vi "phase_one.vi"() -> ()   [LabVIEW 2015]
uses:
  <vilib>/NXT/Block Support/NXT_InputPort.ctl
  <vilib>/NXT/Block Support/NXT_OutputPort.ctl
  <vilib>/NXT/Dual Mode Library/Sound/PlayD.vi
  <vilib>/NXT/Dual Mode Library/Display/clearDisplay.vi
  <vilib>/NXT/Dual Mode Library/Display/drawText.vi
  <vilib>/NXT/Dual Mode Library/Waits/Wait_Num.vi
  <vilib>/NXT/Dual Mode Library/Waits/Wait_Touch.vi
  <vilib>/NXT/Dual Mode Library/Sensors/EV3_Touch_Reset.vi
  <vilib>/NXT/Dual Mode Library/Sensors/Touch_Count.vi
  <vilib>/NXT/Dual Mode Library/Display/drawNumber.vi
  <vilib>/NXT/NXTIO Xnodes/NXTIONodeSubVIs/NXTMotorRunDistance.vi
  <vilib>/NXT/Dual Mode Library/Sensors/EV3_Color_Reflect.vi
  <vilib>/NXT/Dual Mode Library/Display/drawNumber_float.vi
  global1.vi
  <vilib>/NXT/NXTIO Xnodes/AddressXNode/NXTIOAddress.xnode
  <vilib>/NXT/NXTIO Xnodes/NXTIOXNode/NXTIO.xnode
  <vilib>/NXT/Subs/LVHSConnector.ctl
  <vilib>/NXT/LegoClasses/BrickReference/BrickReference.lvclass
panel:
  out "4: Compound 2":string
  out "4: Compound 1":string
  out "3: Compound 1":string
  out "3: Compound 2":string
  out "2: Compound 2":string
  out "1: Compoud 2":string
  out "2: Compound 1":string
  out "1: Compound 1":string
  out "Done with Phase One?":bool
  out "4: Type 2 #":i32
  out "3: Type 2 #":i32
  out "2: Type 2 #":i32
  out "4: Type 1 #":i32
  out "3: Type 1 #":i32
  out "2: Type 1 #":i32
  out "1: Type 2 #":i32
  out "1: Type 1 #":i32
  out "4: Type 2":string
  out "4: Type 1":string
  out "4: Material":string
  out "3: Type 2":string
  out "3: Type 1":string
  out "3: Material":string
  out "2: Type 2":string
  out "2: Type 1":string
  out "2: Material":string
  out "4: 2nd value":i32
  out "3: 2nd value":i32
  out "2: 2nd value":i32
  out "1: 2nd value":i32
  out "4: 1st value":i32
  out "3: 1st value":i32
  out "2: 1st value":i32
  out "1: Type 2":string
  out "1: 1st value":i32
  out "1: Type 1":string
  out "1: Material":string
  out "Times Pressed":i16
  out "4: 2nd num":string
  out "Case 4 bin 2 done?":bool
  out "4: 1st num":string
  out "Case 4 bin 1 done?":bool
  out "3: 2nd num":string
  out "Case 3 bin 2 done?":bool
  out "3: 1st num":string
  out "Case 3 bin 1 done?":bool
  out "2: 2nd num":string
  out "Case 2 bin 2 done?":bool
  out "2: 1st num":string
  out "Case 2 bin 1 done?":bool
  out "1: 2nd num":string
  out "Case 1 bin 2 done?":bool
  out "1: 1st num":string
  out "Case 1 bin 1 done?":bool
  # "Click none = first binary\nClick once = second binary\nClick twice = third binary\nClick thrice = fourth binary\nClick four = conversion menu\nClick five = begin marble operation\nclick 6 + = reset data\n\nFor future final operation, make it case 7 and get \nout of while loop with \"times pressed\" variable hooking up to \noutermost while loop end case."
  # "1) Start the paper on black strip\n2) Tape paper behind strips to make em slightly longer for reading purposes\n3) Use other program for input values, much easier\n4) Motor A = barcode // Port 1 = barcode reader  // Port 2 = touch"
  # "Don't click"
  # "Click once"
  # "Press twice"
  # "Click thrice"
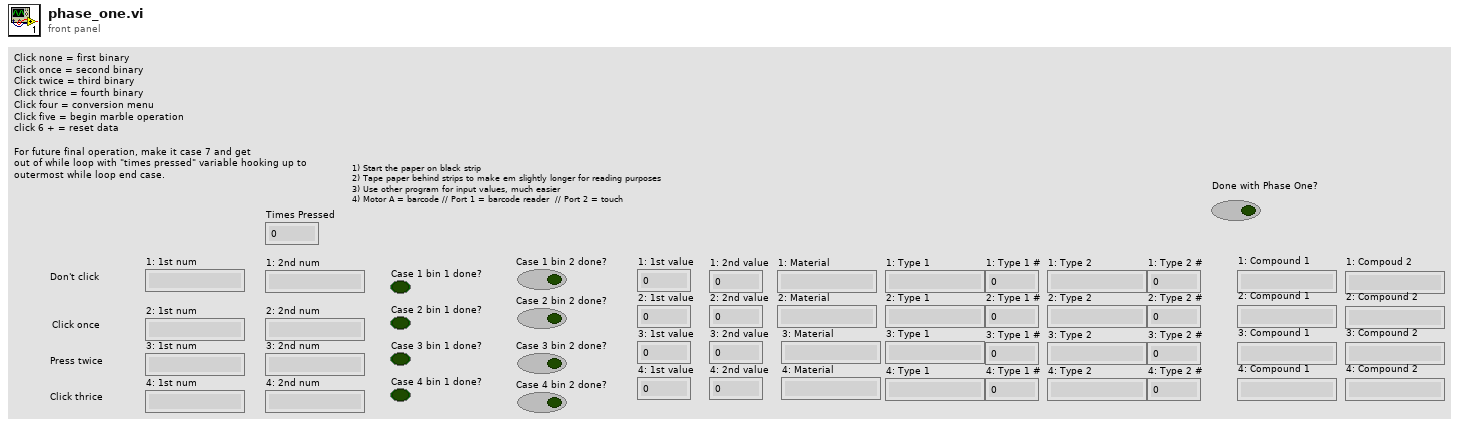
[diagram p1: front panel]
types:
  T1 = typedef "NXT_InputPort.ctl" = u32
  T2 = typedef "LVHSConnector.ctl" = refnum<class "BrickReference.lvclass">
  T3 = typedef "NXT_OutputPort.ctl" = u8
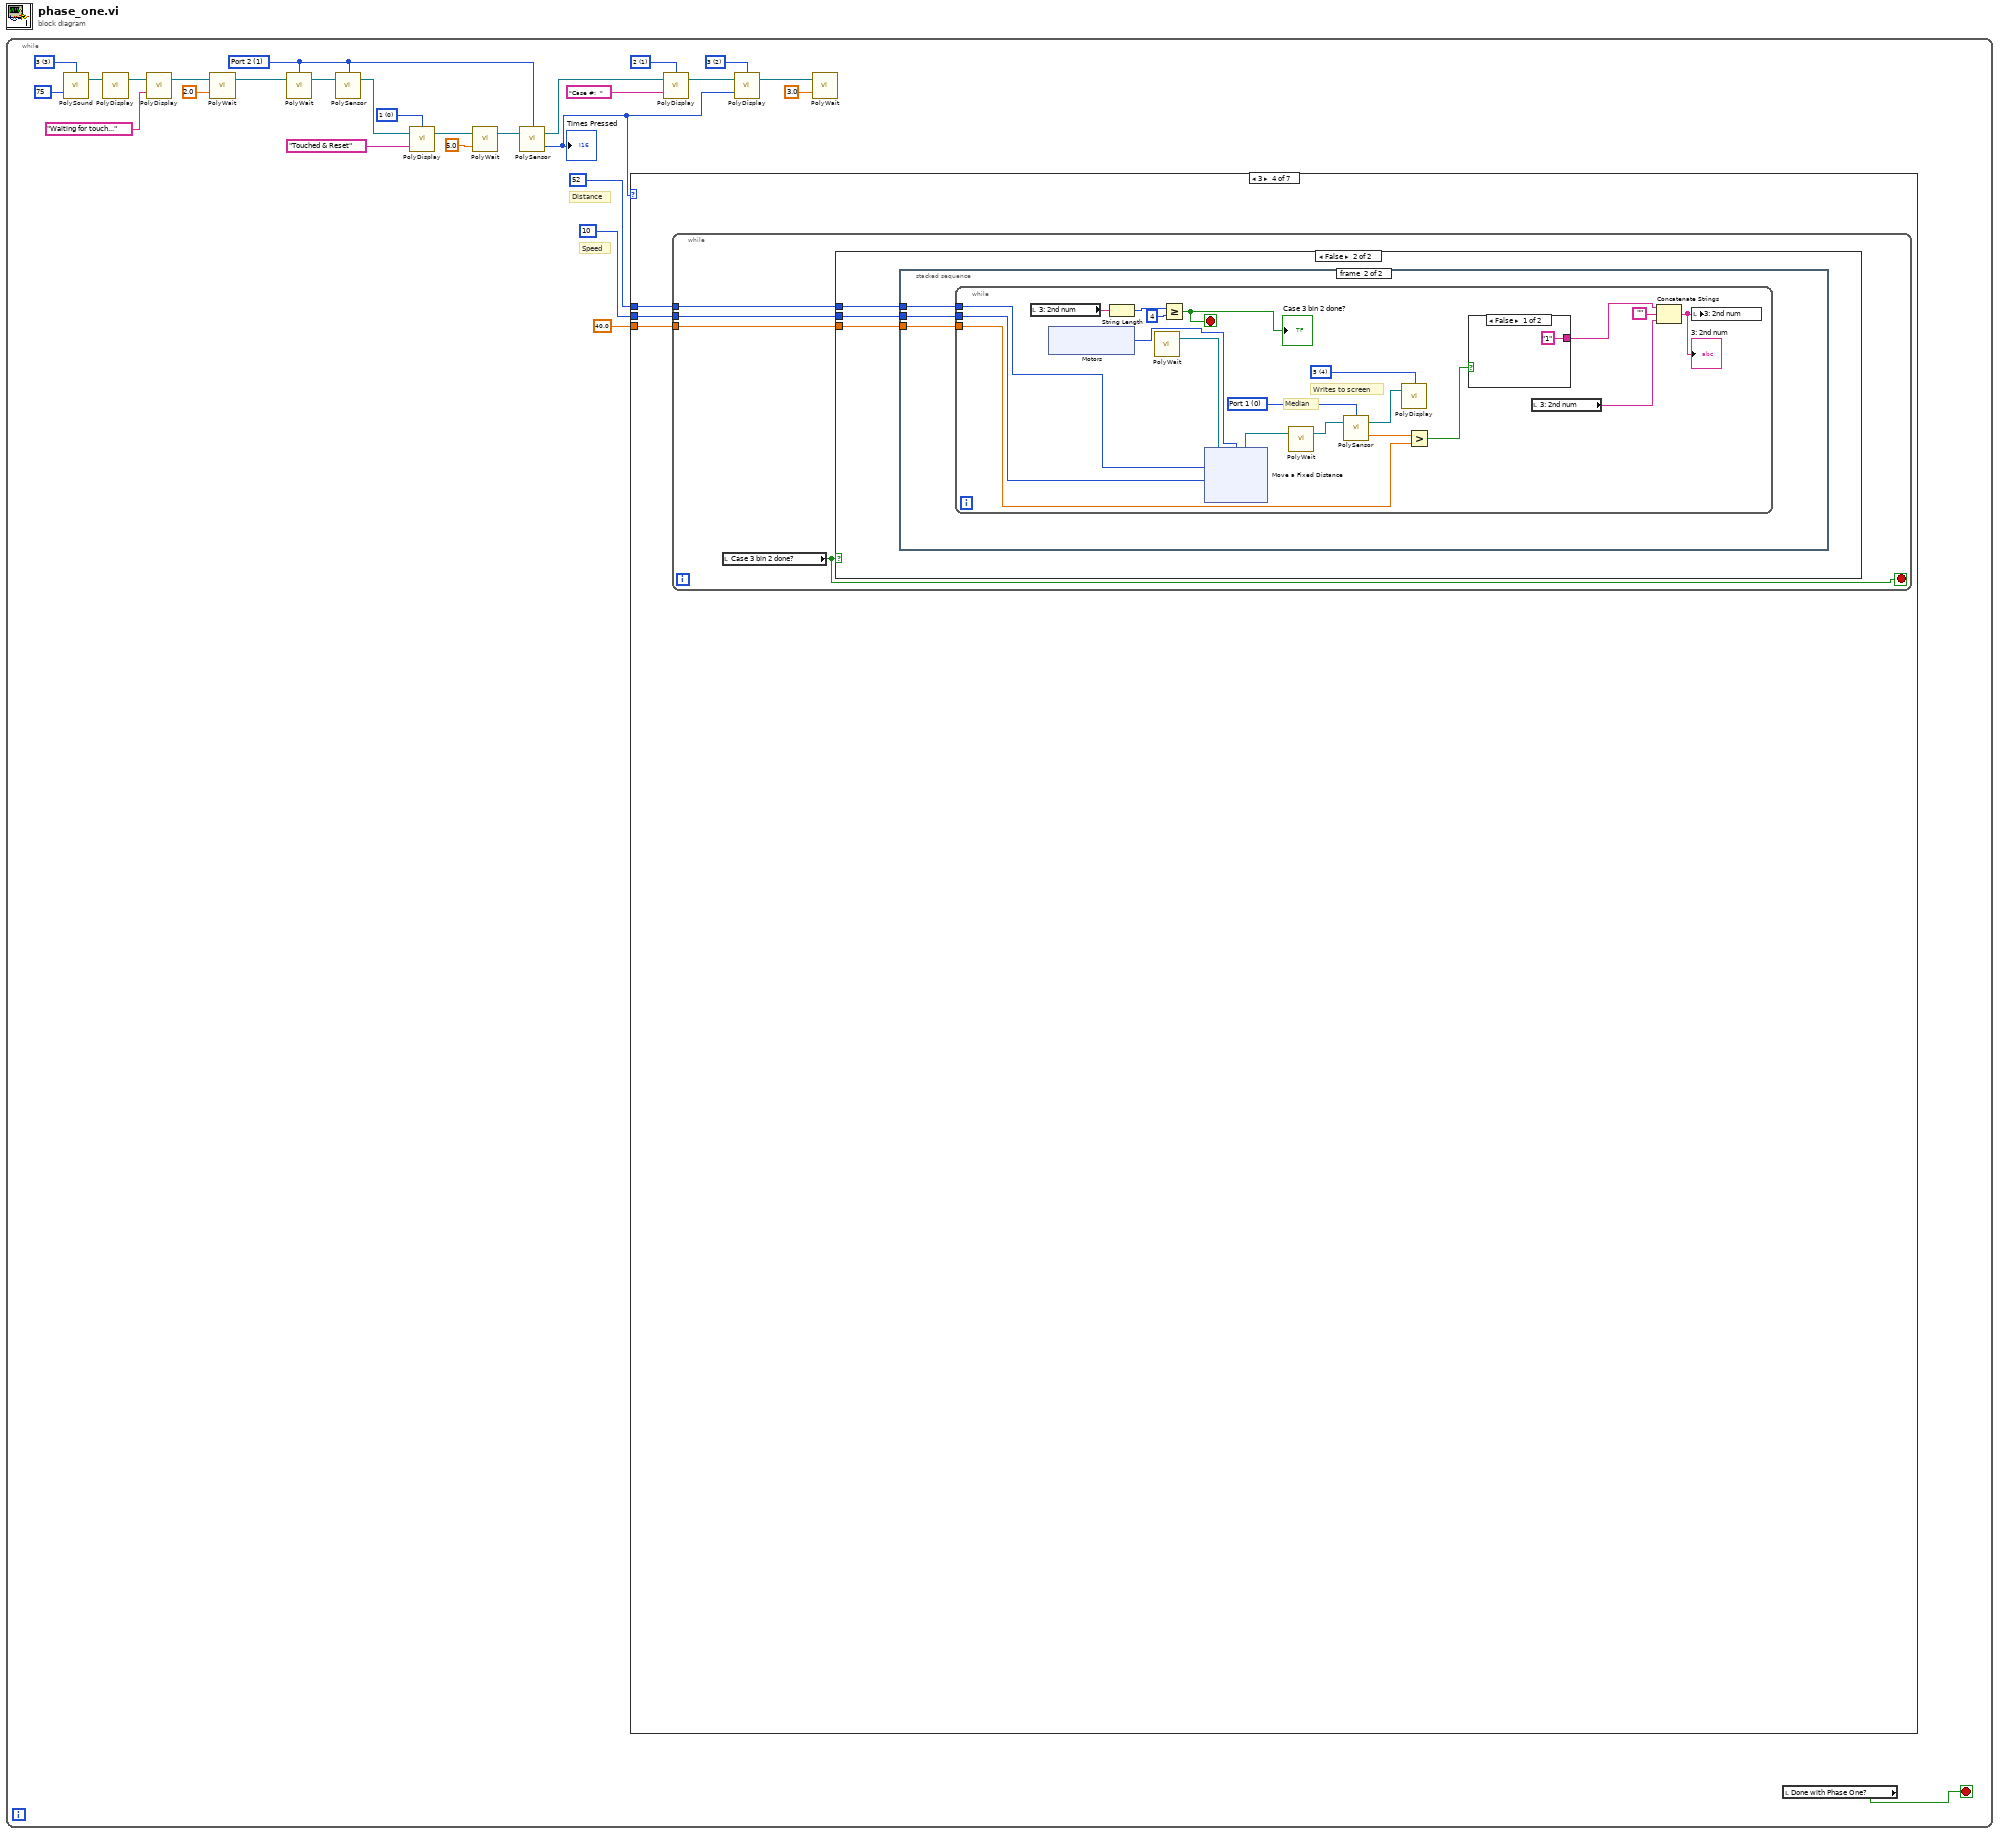
[diagram p0: block diagram]
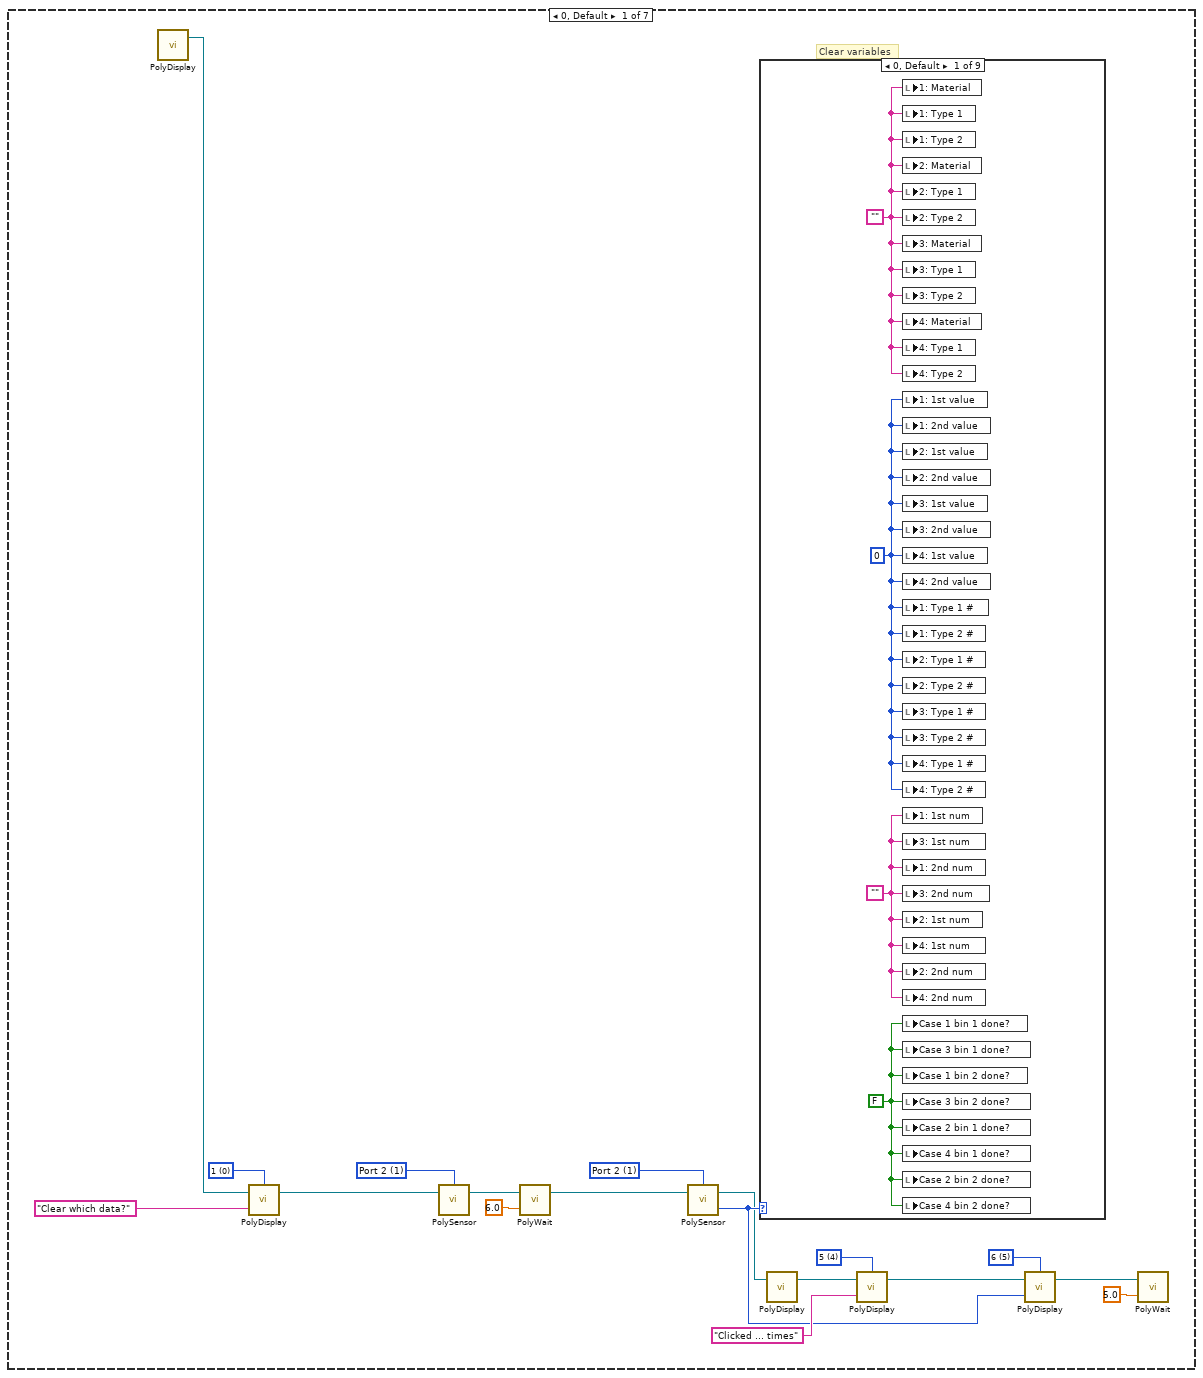
[diagram p2: hidden frame]
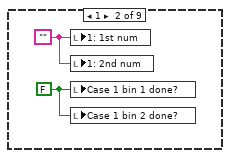
[diagram p3: hidden frame]
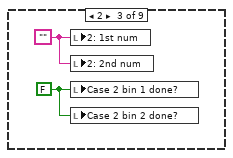
[diagram p4: hidden frame]
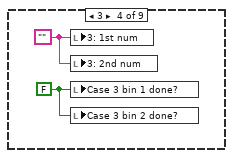
[diagram p5: hidden frame]
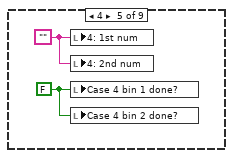
[diagram p6: hidden frame]
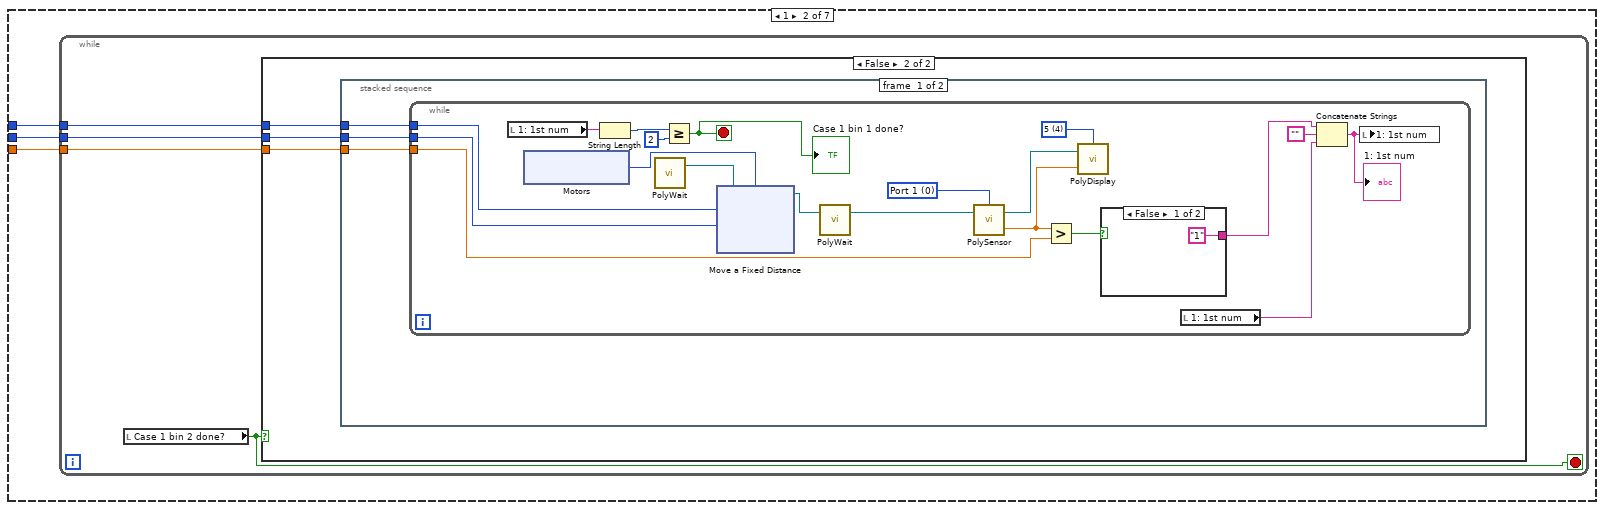
[diagram p11: hidden frame]
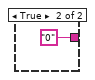
[diagram p13: hidden frame]
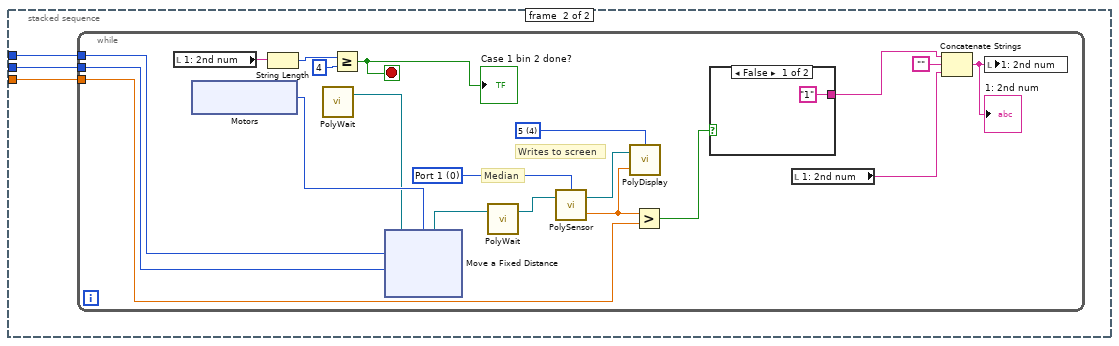
[diagram p14: hidden frame]
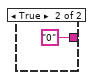
[diagram p15: hidden frame]
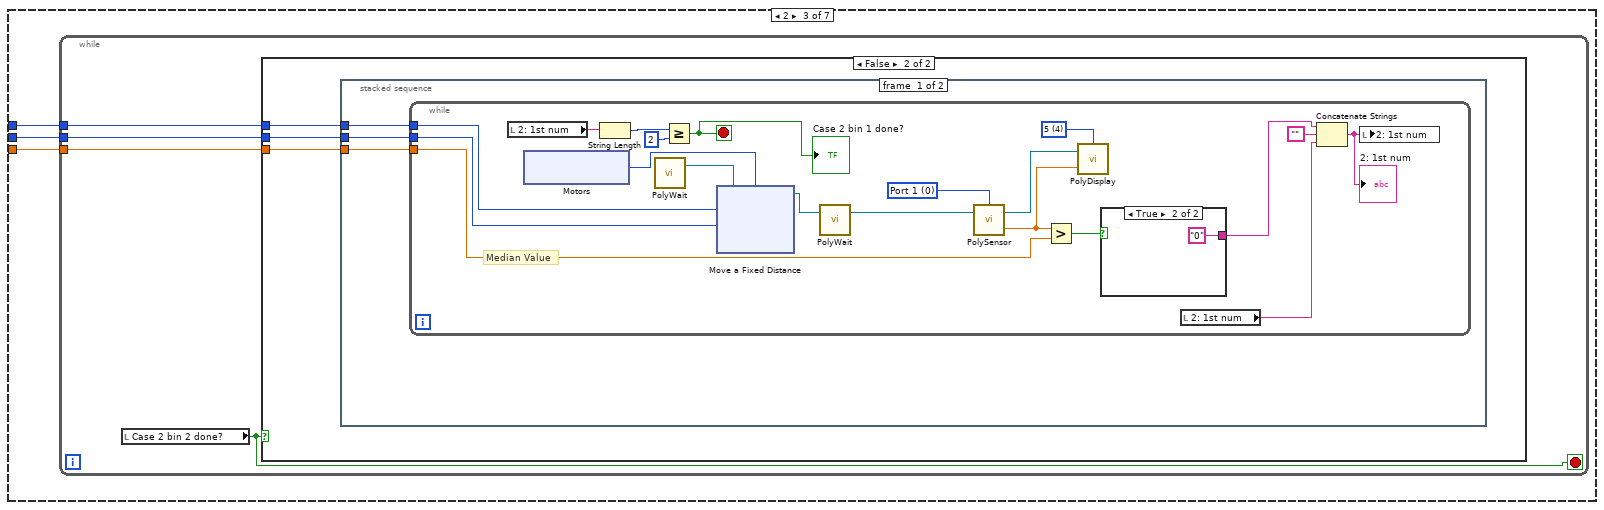
[diagram p16: hidden frame]
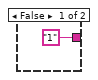
[diagram p18: hidden frame]
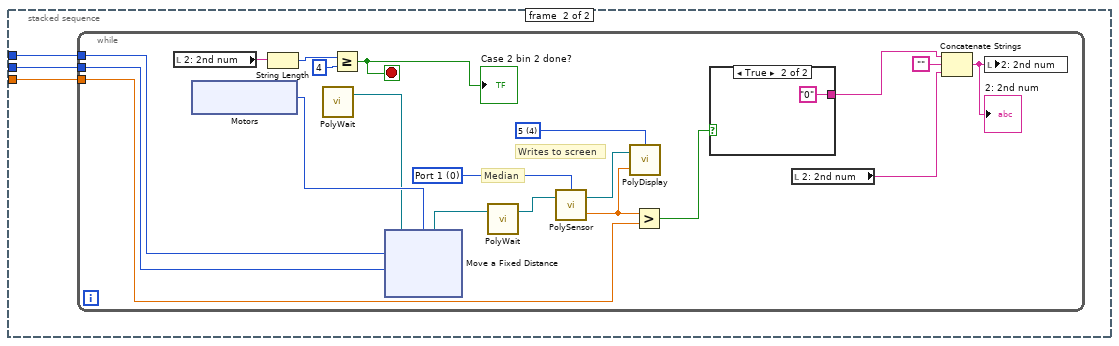
[diagram p19: hidden frame]
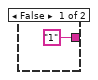
[diagram p20: hidden frame]
diagram:
  n1 = while {
    stop <- w1 stop-if-true
    w5 = u16 3 items=["3"=3, "4"=4, "5"=5, "6"=6, "7"=7] ("Octave")
    w10 = i16 0 items=["1", "2", "3", "4", "5", "6", "7", "8", "9", "10", "11", "12"] ("Line")
    w15 = i16 1 items=["1", "2", "3", "4", "5", "6", "7", "8", "9", "10", "11", "12"] ("Line")
    w24 = i16 2 items=["1", "2", "3", "4", "5", "6", "7", "8", "9", "10", "11", "12"] ("Line")
    w28 = T1 1 items=["Port 1", "Port 2", "Port 3", "Port 4"] ("Port (Port 1)")
    # "Speed"
    # "Distance"
    n2 = call-poly <vilib>:"PolySound.vi"("Duration (500 ms)"=u16 75, "Octave"=w5) -> ("NXT/EV3"=w7:T2)  [unwired: 2 in]
    n3 = call-poly <vilib>:"PolyDisplay.vi"("NXT/EV3"=w7) -> ("NXT/EV3"=w19:T2)  [unwired: 3 in]
    n4 = call-poly <vilib>:"PolyDisplay.vi"("Text"="Waiting for touch...", "NXT/EV3"=w19) -> ("NXT/EV3"=w4:T2)  [unwired: 2 in]
    n5 = call-poly <vilib>:"PolyWait.vi"("Time (1 sec)"=sgl 2.0, "NXT/EV3"=w4) -> ("NXT/EV3"=w3:T2)  [unwired: 2 in]
    n6 = call-poly <vilib>:"PolyWait.vi"("NXT/EV3"=w3, "Port (Port 1)"=w28) -> ("NXT/EV3"=w27:T2)  [unwired: 2 in]
    n7 = call-poly <vilib>:"PolySensor.vi"("NXT/EV3"=w27, "Port (Port 1)"=w28) -> ("NXT/EV3"=w13:T2)  [unwired: 2 in]
    n8 = call-poly <vilib>:"PolyDisplay.vi"("Text"="Touched & Reset", "NXT/EV3"=w13, "Line"=w10) -> ("NXT/EV3"=w11:T2)  [unwired: 1 in]
    n9 = call-poly <vilib>:"PolyWait.vi"("Time (1 sec)"=sgl 5.0, "NXT/EV3"=w11) -> ("NXT/EV3"=w22:T2)  [unwired: 2 in]
    n10 = call-poly <vilib>:"PolySensor.vi"("NXT/EV3"=w22, "Port (Port 1)"=w28) -> ("Count"=w25:i16, "NXT/EV3"=w18:T2)  [unwired: 1 in]
    "Times Pressed" <- w25
    n11 = case shown="3" w25 {
      tunnel: 52 ("Distance 1") -> [_ w61 w143 w225 w307 _ _]
      tunnel: i8 10 ("Power/Speed 1") -> [_ w60 w142 w224 w306 _ _]
      tunnel: sgl 40.0 ("x") -> [_ w59 w141 w223 w305 _ _]
      frame 0, Default {
        w31 = T1 1 items=["Port 1", "Port 2", "Port 3", "Port 4"] ("Port (Port 1)")
        w32 = i16 5 items=["1", "2", "3", "4", "5", "6", "7", "8", "9", "10", "11", "12"] ("Line")
        w37 = T1 1 items=["Port 1", "Port 2", "Port 3", "Port 4"] ("Port (Port 1)")
        w39 = i16 4 items=["1", "2", "3", "4", "5", "6", "7", "8", "9", "10", "11", "12"] ("Line")
        w44 = i16 0 items=["1", "2", "3", "4", "5", "6", "7", "8", "9", "10", "11", "12"] ("Line")
        # "Clear variables"
        n12 = call-poly <vilib>:"PolyDisplay.vi"() -> ("NXT/EV3"=w45:T2)  [unwired: 4 in]
        n13 = call-poly <vilib>:"PolyDisplay.vi"("Text"="Clear which data?", "NXT/EV3"=w45, "Line"=w44) -> ("NXT/EV3"=w30:T2)  [unwired: 1 in]
        n14 = call-poly <vilib>:"PolySensor.vi"("NXT/EV3"=w30, "Port (Port 1)"=w31) -> ("NXT/EV3"=w29:T2)  [unwired: 2 in]
        n15 = call-poly <vilib>:"PolyWait.vi"("Time (1 sec)"=sgl 6.0, "NXT/EV3"=w29) -> ("NXT/EV3"=w42:T2)  [unwired: 2 in]
        n16 = call-poly <vilib>:"PolySensor.vi"("NXT/EV3"=w42, "Port (Port 1)"=w37) -> ("Count"=w38:i16, "NXT/EV3"=w34:T2)  [unwired: 1 in]
        n17 = case shown="0, Default" w38 {
          frame 0, Default {
            w48 = ""
            w49 = 0
            w47 = FALSE
            w50 = ""
            n18 = local write "1: Material"(w48) -> ()
            n19 = local write "1: Type 1"(w48) -> ()
            n20 = local write "1: Type 2"(w48) -> ()
            n21 = local write "2: Material"(w48) -> ()
            n22 = local write "2: Type 1"(w48) -> ()
            n23 = local write "2: Type 2"(w48) -> ()
            n24 = local write "3: Material"(w48) -> ()
            n25 = local write "3: Type 1"(w48) -> ()
            n26 = local write "3: Type 2"(w48) -> ()
            n27 = local write "4: Material"(w48) -> ()
            n28 = local write "4: Type 1"(w48) -> ()
            n29 = local write "4: Type 2"(w48) -> ()
            n30 = local write "1: 1st value"(w49) -> ()
            n31 = local write "1: 2nd value"(w49) -> ()
            n32 = local write "2: 1st value"(w49) -> ()
            n33 = local write "2: 2nd value"(w49) -> ()
            n34 = local write "3: 1st value"(w49) -> ()
            n35 = local write "3: 2nd value"(w49) -> ()
            n36 = local write "4: 1st value"(w49) -> ()
            n37 = local write "4: 2nd value"(w49) -> ()
            n38 = local write "1: Type 1 #"(w49) -> ()
            n39 = local write "1: Type 2 #"(w49) -> ()
            n40 = local write "2: Type 1 #"(w49) -> ()
            n41 = local write "2: Type 2 #"(w49) -> ()
            n42 = local write "3: Type 1 #"(w49) -> ()
            n43 = local write "3: Type 2 #"(w49) -> ()
            n44 = local write "4: Type 1 #"(w49) -> ()
            n45 = local write "4: Type 2 #"(w49) -> ()
            n46 = local write "1: 1st num"(w50) -> ()
            n47 = local write "3: 1st num"(w50) -> ()
            n48 = local write "1: 2nd num"(w50) -> ()
            n49 = local write "3: 2nd num"(w50) -> ()
            n50 = local write "2: 1st num"(w50) -> ()
            n51 = local write "4: 1st num"(w50) -> ()
            n52 = local write "2: 2nd num"(w50) -> ()
            n53 = local write "4: 2nd num"(w50) -> ()
            n54 = local write "Case 1 bin 1 done?"(w47) -> ()
            n55 = local write "Case 3 bin 1 done?"(w47) -> ()
            n56 = local write "Case 1 bin 2 done?"(w47) -> ()
            n57 = local write "Case 3 bin 2 done?"(w47) -> ()
            n58 = local write "Case 2 bin 1 done?"(w47) -> ()
            n59 = local write "Case 4 bin 1 done?"(w47) -> ()
            n60 = local write "Case 2 bin 2 done?"(w47) -> ()
            n61 = local write "Case 4 bin 2 done?"(w47) -> ()
          }
          frame 1 {
            w52 = FALSE
            w51 = ""
            n62 = local write "1: 1st num"(w51) -> ()
            n63 = local write "1: 2nd num"(w51) -> ()
            n64 = local write "Case 1 bin 1 done?"(w52) -> ()
            n65 = local write "Case 1 bin 2 done?"(w52) -> ()
          }
          frame 2 {
            w53 = FALSE
            w54 = ""
            n66 = local write "2: 1st num"(w54) -> ()
            n67 = local write "2: 2nd num"(w54) -> ()
            n68 = local write "Case 2 bin 1 done?"(w53) -> ()
            n69 = local write "Case 2 bin 2 done?"(w53) -> ()
          }
          frame 3 {
            w55 = ""
            w56 = FALSE
            n70 = local write "3: 1st num"(w55) -> ()
            n71 = local write "3: 2nd num"(w55) -> ()
            n72 = local write "Case 3 bin 1 done?"(w56) -> ()
            n73 = local write "Case 3 bin 2 done?"(w56) -> ()
          }
          frame 4 {
            w57 = ""
            w58 = FALSE
            n74 = local write "4: 1st num"(w57) -> ()
            n75 = local write "4: 2nd num"(w57) -> ()
            n76 = local write "Case 4 bin 1 done?"(w58) -> ()
            n77 = local write "Case 4 bin 2 done?"(w58) -> ()
          }
          frame 5 {
            # "Do nothing"
          }
          frame 6 {
            # "Do nothing"
          }
          frame 7 {
            # "Do nothing"
          }
          frame 8 {
            # "Do nothing"
          }
        }
        n78 = call-poly <vilib>:"PolyDisplay.vi"("NXT/EV3"=w34) -> ("NXT/EV3"=w33:T2)  [unwired: 3 in]
        n79 = call-poly <vilib>:"PolyDisplay.vi"("Text"="Clicked ... times", "NXT/EV3"=w33, "Line"=w39) -> ("NXT/EV3"=w36:T2)  [unwired: 1 in]
        n80 = call-poly <vilib>:"PolyDisplay.vi"("number"=w38, "NXT/EV3"=w36, "Line"=w32) -> ("NXT/EV3"=w35:T2)  [unwired: 1 in]
        n81 = call-poly <vilib>:"PolyWait.vi"("Time (1 sec)"=sgl 5.0, "NXT/EV3"=w35) -> ()  [unwired: 2 in, 1 out]
      }
      frame 1 {
        n82 = while {
          tunnel: w61 -> [w65]
          tunnel: w60 -> [w64]
          tunnel: w59 -> [w63]
          stop <- w62 stop-if-true
          n83 = local read "Case 1 bin 2 done?"() -> (w62:bool)
          n84 = case shown="False" w62 {
            tunnel: w65 -> [_ w68]
            tunnel: w64 -> [_ w67]
            tunnel: w63 -> [_ w66]
            frame True {
            }
            frame False {
              n85 = stacked-sequence {
                tunnel: w68 -> [w71 w107]
                tunnel: w67 -> [w70 w106]
                tunnel: w66 -> [w69 w105]
                frame #0 {
                  n86 = while {
                    tunnel: w71 -> [w77]
                    tunnel: w70 -> [w76]
                    tunnel: w69 -> [w75]
                    stop <- w80 stop-if-true
                    w79 = i16 4 items=["1", "2", "3", "4", "5", "6", "7", "8", "9", "10", "11", "12"] ("Line")
                    w90 = T1 0 items=["Port 1", "Port 2", "Port 3", "Port 4"] ("Port (Port 3)")
                    n87 = local read "1: 1st num"() -> (w82:string)
                    n88 = xnode "Motors"() -> ("Motor"=w91:T3)
                    n89 = String Length(string=w82) -> (length=w81:i32)
                    n90 = call-poly <vilib>:"PolyWait.vi"() -> ("NXT/EV3"=w78:T2)  [unwired: 4 in]
                    n91 = Greater Or Equal?(x=w81, y=2) -> (x >= y?=w80:bool)
                    "Case 1 bin 1 done?" <- w80
                    n92 = xnode "Move a Fixed Distance"("Speed 1"=w76, "Distance 1"=w77, "Motors"=w91, "NXT/EV3"=w78) -> ("NXT/EV3"=w89:T2)
                    n93 = call-poly <vilib>:"PolyWait.vi"("NXT/EV3"=w89) -> ("NXT/EV3"=w88:T2)  [unwired: 3 in]
                    n94 = call-poly <vilib>:"PolySensor.vi"("NXT/EV3"=w88, "Port (Port 1)"=w90) -> ("Scaled Value"=w74:sgl, "NXT/EV3"=w73:T2)  [unwired: 1 in]
                    n95 = Greater?(x=w74, y=w75) -> (0:w85:bool)
                    n96 = call-poly <vilib>:"PolyDisplay.vi"("number"=w74, "NXT/EV3"=w73, "Line"=w79) -> ()  [unwired: 1 in, 1 out]
                    n97 = case shown="False" w85 {
                      tunnel: ["1" "0"] -> w87
                      frame False {
                      }
                      frame True {
                      }
                    }
                    n98 = local read "1: 1st num"() -> (w83:string)
                    n99 = Concatenate Strings(w87, "", w83) -> (w84:string)
                    "1: 1st num" <- w84
                    n100 = local write "1: 1st num"(w84) -> ()
                  }
                }
                frame #1 {
                  n101 = while {
                    tunnel: w107 -> [w113]
                    tunnel: w106 -> [w112]
                    tunnel: w105 -> [w111]
                    stop <- w116 stop-if-true
                    w114 = i16 4 items=["1", "2", "3", "4", "5", "6", "7", "8", "9", "10", "11", "12"] ("Line")
                    w126 = T1 0 items=["Port 1", "Port 2", "Port 3", "Port 4"] ("Port (Port 3)")
                    # "Writes to screen"
                    # "Median"
                    n102 = local read "1: 2nd num"() -> (w118:string)
                    n103 = xnode "Motors"() -> ("Motor"=w127:T3)
                    n104 = String Length(string=w118) -> (length=w117:i32)
                    n105 = call-poly <vilib>:"PolyWait.vi"() -> ("NXT/EV3"=w115:T2)  [unwired: 4 in]
                    n106 = Greater Or Equal?(x=w117, y=4) -> (x >= y?=w116:bool)
                    "Case 1 bin 2 done?" <- w116
                    n107 = xnode "Move a Fixed Distance"("Speed 1"=w112, "Distance 1"=w113, "Motors"=w127, "NXT/EV3"=w115) -> ("NXT/EV3"=w125:T2)
                    n108 = call-poly <vilib>:"PolyWait.vi"("NXT/EV3"=w125) -> ("NXT/EV3"=w124:T2)  [unwired: 3 in]
                    n109 = call-poly <vilib>:"PolySensor.vi"("NXT/EV3"=w124, "Port (Port 1)"=w126) -> ("Scaled Value"=w110:sgl, "NXT/EV3"=w109:T2)  [unwired: 1 in]
                    n110 = call-poly <vilib>:"PolyDisplay.vi"("number"=w110, "NXT/EV3"=w109, "Line"=w114) -> ()  [unwired: 1 in, 1 out]
                    n111 = Greater?(x=w110, y=w111) -> (0:w121:bool)
                    n112 = case shown="False" w121 {
                      tunnel: ["1" "0"] -> w123
                      frame False {
                      }
                      frame True {
                      }
                    }
                    n113 = local read "1: 2nd num"() -> (w119:string)
                    n114 = Concatenate Strings(w123, "", w119) -> (w120:string)
                    "1: 2nd num" <- w120
                    n115 = local write "1: 2nd num"(w120) -> ()
                  }
                }
              }
            }
          }
        }
      }
      frame 2 {
        n116 = while {
          tunnel: w143 -> [w147]
          tunnel: w142 -> [w146]
          tunnel: w141 -> [w145]
          stop <- w144 stop-if-true
          n117 = local read "Case 2 bin 2 done?"() -> (w144:bool)
          n118 = case shown="False" w144 {
            tunnel: w147 -> [_ w150]
            tunnel: w146 -> [_ w149]
            tunnel: w145 -> [_ w148]
            frame True {
            }
            frame False {
              n119 = stacked-sequence {
                tunnel: w150 -> [w153 w189]
                tunnel: w149 -> [w152 w188]
                tunnel: w148 -> [w151 w187]
                frame #0 {
                  n120 = while {
                    tunnel: w153 -> [w158]
                    tunnel: w152 -> [w157]
                    tunnel: w151 -> [w156]
                    stop <- w161 stop-if-true
                    w160 = i16 4 items=["1", "2", "3", "4", "5", "6", "7", "8", "9", "10", "11", "12"] ("Line")
                    w172 = T1 0 items=["Port 1", "Port 2", "Port 3", "Port 4"] ("Port (Port 3)")
                    # "Median Value"
                    n121 = local read "2: 1st num"() -> (w164:string)
                    n122 = xnode "Motors"() -> ("Motor"=w173:T3)
                    n123 = String Length(string=w164) -> (length=w163:i32)
                    n124 = call-poly <vilib>:"PolyWait.vi"() -> ("NXT/EV3"=w159:T2)  [unwired: 4 in]
                    n125 = Greater Or Equal?(x=w163, y=2) -> (x >= y?=w161:bool)
                    "Case 2 bin 1 done?" <- w161
                    n126 = xnode "Move a Fixed Distance"("Speed 1"=w157, "Distance 1"=w158, "Motors"=w173, "NXT/EV3"=w159) -> ("NXT/EV3"=w171:T2)
                    n127 = call-poly <vilib>:"PolyWait.vi"("NXT/EV3"=w171) -> ("NXT/EV3"=w170:T2)  [unwired: 3 in]
                    n128 = call-poly <vilib>:"PolySensor.vi"("NXT/EV3"=w170, "Port (Port 1)"=w172) -> ("Scaled Value"=w155:sgl, "NXT/EV3"=w154:T2)  [unwired: 1 in]
                    n129 = Greater?(x=w155, y=w156) -> (0:w167:bool)
                    n130 = call-poly <vilib>:"PolyDisplay.vi"("number"=w155, "NXT/EV3"=w154, "Line"=w160) -> ()  [unwired: 1 in, 1 out]
                    n131 = case shown="True" w167 {
                      tunnel: ["1" "0"] -> w169
                      frame False {
                      }
                      frame True {
                      }
                    }
                    n132 = local read "2: 1st num"() -> (w165:string)
                    n133 = Concatenate Strings(w169, "", w165) -> (w166:string)
                    "2: 1st num" <- w166
                    n134 = local write "2: 1st num"(w166) -> ()
                  }
                }
                frame #1 {
                  n135 = while {
                    tunnel: w189 -> [w194]
                    tunnel: w188 -> [w193]
                    tunnel: w187 -> [w192]
                    stop <- w197 stop-if-true
                    w195 = i16 4 items=["1", "2", "3", "4", "5", "6", "7", "8", "9", "10", "11", "12"] ("Line")
                    w208 = T1 0 items=["Port 1", "Port 2", "Port 3", "Port 4"] ("Port (Port 3)")
                    # "Writes to screen"
                    # "Median"
                    n136 = local read "2: 2nd num"() -> (w200:string)
                    n137 = xnode "Motors"() -> ("Motor"=w209:T3)
                    n138 = String Length(string=w200) -> (length=w199:i32)
                    n139 = call-poly <vilib>:"PolyWait.vi"() -> ("NXT/EV3"=w196:T2)  [unwired: 4 in]
                    n140 = Greater Or Equal?(x=w199, y=4) -> (x >= y?=w197:bool)
                    "Case 2 bin 2 done?" <- w197
                    n141 = xnode "Move a Fixed Distance"("Speed 1"=w193, "Distance 1"=w194, "Motors"=w209, "NXT/EV3"=w196) -> ("NXT/EV3"=w207:T2)
                    n142 = call-poly <vilib>:"PolyWait.vi"("NXT/EV3"=w207) -> ("NXT/EV3"=w206:T2)  [unwired: 3 in]
                    n143 = call-poly <vilib>:"PolySensor.vi"("NXT/EV3"=w206, "Port (Port 1)"=w208) -> ("Scaled Value"=w190:sgl, "NXT/EV3"=w191:T2)  [unwired: 1 in]
                    n144 = call-poly <vilib>:"PolyDisplay.vi"("number"=w190, "NXT/EV3"=w191, "Line"=w195) -> ()  [unwired: 1 in, 1 out]
                    n145 = Greater?(x=w190, y=w192) -> (0:w203:bool)
                    n146 = case shown="True" w203 {
                      tunnel: ["1" "0"] -> w205
                      frame False {
                      }
                      frame True {
                      }
                    }
                    n147 = local read "2: 2nd num"() -> (w201:string)
                    n148 = Concatenate Strings(w205, "", w201) -> (w202:string)
                    "2: 2nd num" <- w202
                    n149 = local write "2: 2nd num"(w202) -> ()
                  }
                }
              }
            }
          }
        }
      }
      frame 3 {
        n150 = while {
          tunnel: w225 -> [w229]
          tunnel: w224 -> [w228]
          tunnel: w223 -> [w227]
          stop <- w226 stop-if-true
          n151 = local read "Case 3 bin 2 done?"() -> (w226:bool)
          n152 = case shown="False" w226 {
            tunnel: w229 -> [_ w232]
            tunnel: w228 -> [_ w231]
            tunnel: w227 -> [_ w230]
            frame True {
            }
            frame False {
              n153 = stacked-sequence {
                tunnel: w232 -> [w235 w270]
                tunnel: w231 -> [w234 w271]
                tunnel: w230 -> [w233 w269]
                frame #0 {
                  n154 = while {
                    tunnel: w235 -> [w240]
                    tunnel: w234 -> [w239]
                    tunnel: w233 -> [w238]
                    stop <- w243 stop-if-true
                    w242 = i16 4 items=["1", "2", "3", "4", "5", "6", "7", "8", "9", "10", "11", "12"] ("Line")
                    w254 = T1 0 items=["Port 1", "Port 2", "Port 3", "Port 4"] ("Port (Port 3)")
                    n155 = local read "3: 1st num"() -> (w246:string)
                    n156 = xnode "Motors"() -> ("Motor"=w255:T3)
                    n157 = String Length(string=w246) -> (length=w245:i32)
                    n158 = call-poly <vilib>:"PolyWait.vi"() -> ("NXT/EV3"=w241:T2)  [unwired: 4 in]
                    n159 = Greater Or Equal?(x=w245, y=2) -> (x >= y?=w243:bool)
                    "Case 3 bin 1 done?" <- w243
                    n160 = xnode "Move a Fixed Distance"("Speed 1"=w239, "Distance 1"=w240, "Motors"=w255, "NXT/EV3"=w241) -> ("NXT/EV3"=w253:T2)
                    n161 = call-poly <vilib>:"PolyWait.vi"("NXT/EV3"=w253) -> ("NXT/EV3"=w252:T2)  [unwired: 3 in]
                    n162 = call-poly <vilib>:"PolySensor.vi"("NXT/EV3"=w252, "Port (Port 1)"=w254) -> ("Scaled Value"=w237:sgl, "NXT/EV3"=w236:T2)  [unwired: 1 in]
                    n163 = Greater?(x=w237, y=w238) -> (0:w249:bool)
                    n164 = call-poly <vilib>:"PolyDisplay.vi"("number"=w237, "NXT/EV3"=w236, "Line"=w242) -> ()  [unwired: 1 in, 1 out]
                    n165 = case shown="False" w249 {
                      tunnel: ["1" "0"] -> w251
                      frame False {
                      }
                      frame True {
                      }
                    }
                    n166 = local read "3: 1st num"() -> (w247:string)
                    n167 = Concatenate Strings(w251, "", w247) -> (w248:string)
                    "3: 1st num" <- w248
                    n168 = local write "3: 1st num"(w248) -> ()
                  }
                }
                frame #1 {
                  n169 = while {
                    tunnel: w271 -> [w272]
                    tunnel: w270 -> [w273]
                    tunnel: w269 -> [w276]
                    stop <- w279 stop-if-true
                    w277 = i16 4 items=["1", "2", "3", "4", "5", "6", "7", "8", "9", "10", "11", "12"] ("Line")
                    w290 = T1 0 items=["Port 1", "Port 2", "Port 3", "Port 4"] ("Port (Port 3)")
                    # "Writes to screen"
                    # "Median"
                    n170 = local read "3: 2nd num"() -> (w282:string)
                    n171 = xnode "Motors"() -> ("Motor"=w291:T3)
                    n172 = String Length(string=w282) -> (length=w281:i32)
                    n173 = call-poly <vilib>:"PolyWait.vi"() -> ("NXT/EV3"=w278:T2)  [unwired: 4 in]
                    n174 = Greater Or Equal?(x=w281, y=4) -> (x >= y?=w279:bool)
                    "Case 3 bin 2 done?" <- w279
                    n175 = xnode "Move a Fixed Distance"("Speed 1"=w272, "Distance 1"=w273, "Motors"=w291, "NXT/EV3"=w278) -> ("NXT/EV3"=w289:T2)
                    n176 = call-poly <vilib>:"PolyWait.vi"("NXT/EV3"=w289) -> ("NXT/EV3"=w288:T2)  [unwired: 3 in]
                    n177 = call-poly <vilib>:"PolySensor.vi"("NXT/EV3"=w288, "Port (Port 1)"=w290) -> ("Scaled Value"=w275:sgl, "NXT/EV3"=w274:T2)  [unwired: 1 in]
                    n178 = call-poly <vilib>:"PolyDisplay.vi"("NXT/EV3"=w274, "Line"=w277) -> ()  [unwired: 2 in, 1 out]
                    n179 = Greater?(x=w275, y=w276) -> (0:w285:bool)
                    n180 = case shown="False" w285 {
                      tunnel: ["1" "0"] -> w287
                      frame False {
                      }
                      frame True {
                      }
                    }
                    n181 = local read "3: 2nd num"() -> (w283:string)
                    n182 = Concatenate Strings(w287, "", w283) -> (w284:string)
                    "3: 2nd num" <- w284
                    n183 = local write "3: 2nd num"(w284) -> ()
                  }
                }
              }
            }
          }
        }
      }
      frame 4 {
        n184 = while {
          tunnel: w307 -> [w311]
          tunnel: w306 -> [w310]
          tunnel: w305 -> [w309]
          stop <- w308 stop-if-true
          n185 = local read "Case 4 bin 2 done?"() -> (w308:bool)
          n186 = case shown="False" w308 {
            tunnel: w311 -> [_ w314]
            tunnel: w310 -> [_ w313]
            tunnel: w309 -> [_ w312]
            frame True {
            }
            frame False {
              n187 = stacked-sequence {
                tunnel: w314 -> [w317 w353]
                tunnel: w313 -> [w316 w352]
                tunnel: w312 -> [w315 w351]
                frame #0 {
                  n188 = while {
                    tunnel: w317 -> [w322]
                    tunnel: w316 -> [w321]
                    tunnel: w315 -> [w320]
                    stop <- w325 stop-if-true
                    w324 = i16 4 items=["1", "2", "3", "4", "5", "6", "7", "8", "9", "10", "11", "12"] ("Line")
                    w336 = T1 0 items=["Port 1", "Port 2", "Port 3", "Port 4"] ("Port (Port 3)")
                    n189 = local read "4: 1st num"() -> (w328:string)
                    n190 = xnode "Motors"() -> ("Motor"=w337:T3)
                    n191 = String Length(string=w328) -> (length=w327:i32)
                    n192 = call-poly <vilib>:"PolyWait.vi"() -> ("NXT/EV3"=w323:T2)  [unwired: 4 in]
                    n193 = Greater Or Equal?(x=w327, y=2) -> (x >= y?=w325:bool)
                    "Case 4 bin 1 done?" <- w325
                    n194 = xnode "Move a Fixed Distance"("Speed 1"=w321, "Distance 1"=w322, "Motors"=w337, "NXT/EV3"=w323) -> ("NXT/EV3"=w335:T2)
                    n195 = call-poly <vilib>:"PolyWait.vi"("NXT/EV3"=w335) -> ("NXT/EV3"=w334:T2)  [unwired: 3 in]
                    n196 = call-poly <vilib>:"PolySensor.vi"("NXT/EV3"=w334, "Port (Port 1)"=w336) -> ("Scaled Value"=w319:sgl, "NXT/EV3"=w318:T2)  [unwired: 1 in]
                    n197 = Greater?(x=w319, y=w320) -> (0:w331:bool)
                    n198 = call-poly <vilib>:"PolyDisplay.vi"("number"=w319, "NXT/EV3"=w318, "Line"=w324) -> ()  [unwired: 1 in, 1 out]
                    n199 = case shown="False" w331 {
                      tunnel: ["1" "0"] -> w333
                      frame False {
                      }
                      frame True {
                      }
                    }
                    n200 = local read "4: 1st num"() -> (w329:string)
                    n201 = Concatenate Strings(w333, "", w329) -> (w330:string)
                    "4: 1st num" <- w330
                    n202 = local write "4: 1st num"(w330) -> ()
                  }
                }
                frame #1 {
                  n203 = while {
                    tunnel: w353 -> [w358]
                    tunnel: w352 -> [w357]
                    tunnel: w351 -> [w356]
                    stop <- w361 stop-if-true
                    w359 = i16 4 items=["1", "2", "3", "4", "5", "6", "7", "8", "9", "10", "11", "12"] ("Line")
                    w372 = T1 0 items=["Port 1", "Port 2", "Port 3", "Port 4"] ("Port (Port 3)")
                    n204 = local read "4: 2nd num"() -> (w364:string)
                    n205 = xnode "Motors"() -> ("Motor"=w373:T3)
                    n206 = String Length(string=w364) -> (length=w363:i32)
                    n207 = call-poly <vilib>:"PolyWait.vi"() -> ("NXT/EV3"=w360:T2)  [unwired: 4 in]
                    n208 = Greater Or Equal?(x=w363, y=4) -> (x >= y?=w361:bool)
                    "Case 4 bin 2 done?" <- w361
                    n209 = xnode "Move a Fixed Distance"("Speed 1"=w357, "Distance 1"=w358, "Motors"=w373, "NXT/EV3"=w360) -> ("NXT/EV3"=w371:T2)
                    n210 = call-poly <vilib>:"PolyWait.vi"("NXT/EV3"=w371) -> ("NXT/EV3"=w370:T2)  [unwired: 3 in]
                    n211 = call-poly <vilib>:"PolySensor.vi"("NXT/EV3"=w370, "Port (Port 1)"=w372) -> ("Scaled Value"=w355:sgl, "NXT/EV3"=w354:T2)  [unwired: 1 in]
                    n212 = Greater?(x=w355, y=w356) -> (0:w367:bool)
                    n213 = call-poly <vilib>:"PolyDisplay.vi"("number"=w355, "NXT/EV3"=w354, "Line"=w359) -> ()  [unwired: 1 in, 1 out]
                    n214 = case shown="True" w367 {
                      tunnel: ["1" "0"] -> w369
                      frame False {
                      }
                      frame True {
                      }
                    }
                    n215 = local read "4: 2nd num"() -> (w365:string)
                    n216 = Concatenate Strings(w369, "", w365) -> (w366:string)
                    "4: 2nd num" <- w366
                    n217 = local write "4: 2nd num"(w366) -> ()
                  }
                }
              }
            }
          }
        }
      }
      frame 5 {
        w390 = i16 2 items=["1", "2", "3", "4", "5", "6", "7", "8", "9", "10", "11", "12"] ("Line")
        n218 = local read "4: 2nd value"() -> (w392:i32)
        n219 = local read "3: 2nd value"() -> (w393:i32)
        n220 = local read "2: 2nd value"() -> (w394:i32)
        n221 = local read "1: 2nd value"() -> (w402:i32)
        n222 = local read "3: 2nd num"() -> (w410:string)
        n223 = local read "1: 1st value"() -> (w407:i32)
        n224 = local read "2: 1st value"() -> (w406:i32)
        n225 = local read "3: 1st value"() -> (w405:i32)
        n226 = local read "4: 1st value"() -> (w404:i32)
        n227 = local read "4: 2nd num"() -> (w411:string)
        n228 = local read "4: 1st num"() -> (w420:string)
        n229 = local read "3: 1st num"() -> (w419:string)
        n230 = local read "2: 2nd num"() -> (w409:string)
        n231 = local read "1: 2nd num"() -> (w408:string)
        n232 = local read "2: 1st num"() -> (w418:string)
        n233 = local read "1: 1st num"() -> (w416:string)
        n234 = case shown="10" w392 {
          tunnel: [0 1 2 3 0 1 2 3 0 1 2 3 0 1 2 3] -> w396
          tunnel: [0 0 0 0 1 1 1 1 2 2 2 2 3 3 3 3] -> w395
          frame 1, Default {
          }
          frame 10 {
          }
          frame 11 {
          }
          frame 100 {
          }
          frame 101 {
          }
          frame 110 {
          }
          frame 111 {
          }
          frame 1000 {
          }
          frame 1001 {
          }
          frame 1010 {
          }
          frame 1011 {
          }
          frame 1100 {
          }
          frame 1101 {
          }
          frame 1110 {
          }
          frame 1111 {
          }
          frame 10000 {
          }
        }
        "4: Type 1 #" <- w396
        "4: Type 2 #" <- w395
        n235 = case shown="10" w393 {
          tunnel: [0 1 2 3 0 1 2 3 0 1 2 3 0 1 2 3] -> w398
          tunnel: [0 0 0 0 1 1 1 1 2 2 2 2 3 3 3 3] -> w397
          frame 1, Default {
          }
          frame 10 {
          }
          frame 11 {
          }
          frame 100 {
          }
          frame 101 {
          }
          frame 110 {
          }
          frame 111 {
          }
          frame 1000 {
          }
          frame 1001 {
          }
          frame 1010 {
          }
          frame 1011 {
          }
          frame 1100 {
          }
          frame 1101 {
          }
          frame 1110 {
          }
          frame 1111 {
          }
          frame 10000 {
          }
        }
        "3: Type 1 #" <- w398
        "3: Type 2 #" <- w397
        n236 = case shown="10" w394 {
          tunnel: [0 1 2 3 0 1 2 3 0 1 2 3 0 1 2 3] -> w400
          tunnel: [0 0 0 0 1 1 1 1 2 2 2 2 3 3 3 3] -> w399
          frame 1, Default {
          }
          frame 10 {
          }
          frame 11 {
          }
          frame 100 {
          }
          frame 101 {
          }
          frame 110 {
          }
          frame 111 {
          }
          frame 1000 {
          }
          frame 1001 {
          }
          frame 1010 {
          }
          frame 1011 {
          }
          frame 1100 {
          }
          frame 1101 {
          }
          frame 1110 {
          }
          frame 1111 {
          }
          frame 10000 {
          }
        }
        "2: Type 1 #" <- w400
        "2: Type 2 #" <- w399
        n237 = case shown="10" w402 {
          tunnel: [0 1 2 3 0 1 2 3 0 1 2 3 0 1 2 3] -> w403
          tunnel: [0 0 0 0 1 1 1 1 2 2 2 2 3 3 3 3] -> w401
          frame 1, Default {
          }
          frame 10 {
          }
          frame 11 {
          }
          frame 100 {
          }
          frame 101 {
          }
          frame 110 {
          }
          frame 111 {
          }
          frame 1000 {
          }
          frame 1001 {
          }
          frame 1010 {
          }
          frame 1011 {
          }
          frame 1100 {
          }
          frame 1101 {
          }
          frame 1110 {
          }
          frame 1111 {
          }
          frame 10000 {
          }
        }
        "1: Type 1 #" <- w403
        "1: Type 2 #" <- w401
        n238 = Decimal String To Number(string=w418) -> (number=→"2: 1st value":i32)  [unwired: 2 in, 1 out]
        n239 = case shown="10" w407 {
          frame 0, Default {
          }
          frame 1 {
            "1: Material" <- "White" ("Material 1")
            "1: Type 1" <- "Large"
            "1: Type 2" <- "Small"
          }
          frame 10 {
            n240 = local write "1: Type 2"("Small") -> ()
            n241 = local write "1: Type 1"("Large") -> ()
            n242 = local write "1: Material"("Red" ("Material 1")) -> ()
          }
          frame 11 {
            n243 = local write "1: Type 2"("Small") -> ()
            n244 = local write "1: Type 1"("Large") -> ()
            n245 = local write "1: Material"("Blue" ("Material 1")) -> ()
          }
          frame 100 {
            n246 = local write "1: Type 1"("Steel") -> ()
            n247 = local write "1: Type 2"("HDPE") -> ()
            n248 = local write "1: Material"("Special") -> ()
          }
        }
        n249 = case shown="100" w406 {
          frame 0, Default {
          }
          frame 1 {
            "2: Material" <- "White" ("Material 1")
            "2: Type 1" <- "Large"
            "2: Type 2" <- "Small"
          }
          frame 10 {
            n250 = local write "2: Type 2"("Small") -> ()
            n251 = local write "2: Type 1"("Large") -> ()
            n252 = local write "2: Material"("Red" ("Material 1")) -> ()
          }
          frame 11 {
            n253 = local write "2: Type 2"("Small") -> ()
            n254 = local write "2: Type 1"("Large") -> ()
            n255 = local write "2: Material"("Blue" ("Material 1")) -> ()
          }
          frame 100 {
            n256 = local write "2: Type 1"("Steel") -> ()
            n257 = local write "2: Type 2"("HDPE") -> ()
            n258 = local write "2: Material"("Special") -> ()
          }
        }
        n259 = case shown="100" w405 {
          frame 0, Default {
          }
          frame 1 {
            "3: Type 2" <- "Small"
            "3: Type 1" <- "Large"
            "3: Material" <- "White" ("Material 1")
          }
          frame 10 {
            n260 = local write "3: Type 2"("Small") -> ()
            n261 = local write "3: Type 1"("Large") -> ()
            n262 = local write "3: Material"("Red" ("Material 1")) -> ()
          }
          frame 11 {
            n263 = local write "3: Type 2"("Small") -> ()
            n264 = local write "3: Type 1"("Large") -> ()
            n265 = local write "3: Material"("Blue" ("Material 1")) -> ()
          }
          frame 100 {
            n266 = local write "3: Type 1"("Steel") -> ()
            n267 = local write "3: Type 2"("HDPE") -> ()
            n268 = local write "3: Material"("Special") -> ()
          }
        }
        n269 = case shown="100" w404 {
          frame 0, Default {
          }
          frame 1 {
            "4: Material" <- "White" ("Material 1")
            "4: Type 1" <- "Large"
            "4: Type 2" <- "Small"
          }
          frame 10 {
            n270 = local write "4: Type 2"("Small") -> ()
            n271 = local write "4: Type 1"("Large") -> ()
            n272 = local write "4: Material"("Red" ("Material 1")) -> ()
          }
          frame 11 {
            n273 = local write "2: Type 2"("Small") -> ()
            n274 = local write "2: Type 1"("Large") -> ()
            n275 = local write "4: Material"("Blue" ("Material 1")) -> ()
          }
          frame 100 {
            n276 = local write "4: Type 1"("Steel") -> ()
            n277 = local write "4: Type 2"("HDPE") -> ()
            n278 = local write "4: Material"("Special") -> ()
          }
        }
        n279 = Decimal String To Number(string=w416) -> (number=→"1: 1st value":i32)  [unwired: 2 in, 1 out]
        n280 = Decimal String To Number(string=w411) -> (number=→"4: 2nd value":i32)  [unwired: 2 in, 1 out]
        n281 = Decimal String To Number(string=w420) -> (number=→"4: 1st value":i32)  [unwired: 2 in, 1 out]
        n282 = Decimal String To Number(string=w410) -> (number=→"3: 2nd value":i32)  [unwired: 2 in, 1 out]
        n283 = Decimal String To Number(string=w419) -> (number=→"3: 1st value":i32)  [unwired: 2 in, 1 out]
        n284 = Decimal String To Number(string=w409) -> (number=→"2: 2nd value":i32)  [unwired: 2 in, 1 out]
        n285 = Decimal String To Number(string=w408) -> (number=→"1: 2nd value":i32)  [unwired: 2 in, 1 out]
        n286 = call-poly <vilib>:"PolyDisplay.vi"() -> ("NXT/EV3"=w389:T2)  [unwired: 4 in]
        n287 = call-poly <vilib>:"PolyDisplay.vi"("Text"="Conversion menu", "NXT/EV3"=w389, "Line"=w390) -> ("NXT/EV3"=w387:T2)  [unwired: 1 in]
        n288 = call-poly <vilib>:"PolyWait.vi"("Time (1 sec)"=sgl 5.0, "NXT/EV3"=w387) -> ()  [unwired: 2 in, 1 out]
      }
      frame 6 {
        # "COMPOUND IDEA"
        n289 = local read "3: Type 1 #"() -> (w623:i32)
        n290 = local read "3: Type 2 #"() -> (w622:i32)
        n291 = local read "4: Type 1 #"() -> (w621:i32)
        n292 = local read "4: Type 2 #"() -> (w620:i32)
        n293 = local read "3: Type 1"() -> (w613:string)
        n294 = local read "3: Type 2"() -> (w609:string)
        n295 = local read "2: Type 1 #"() -> (w625:i32)
        n296 = local read "2: Type 2 #"() -> (w624:i32)
        n297 = local read "4: Type 1"() -> (w612:string)
        n298 = local read "4: Type 2"() -> (w608:string)
        n299 = local read "1: Type 1"() -> (w619:string)
        n300 = local read "1: Type 2"() -> (w611:string)
        n301 = local read "2: Type 1"() -> (w614:string)
        n302 = local read "2: Type 2"() -> (w610:string)
        n303 = local read "1: Type 1 #"() -> (w627:i32)
        n304 = local read "1: Type 2 #"() -> (w626:i32)
        n305 = local read "2: Material"() -> (w617:string)
        n306 = local read "3: Material"() -> (w616:string)
        n307 = local read "1: Material"() -> (w618:string)
        n308 = local read "4: Material"() -> (w615:string)
        n309 = global write "global1.vi" "1: Type 1 #"(w627) -> ()
        n310 = global write "global1.vi" "1: Type 2 #"(w626) -> ()
        n311 = global write "global1.vi" "2: Type 1 #"(w625) -> ()
        n312 = global write "global1.vi" "2: Type 2 #"(w624) -> ()
        n313 = global write "global1.vi" "3: Type 1 #"(w623) -> ()
        n314 = global write "global1.vi" "3: Type 2 #"(w622) -> ()
        n315 = global write "global1.vi" "4: Type 1 #"(w621) -> ()
        n316 = global write "global1.vi" "4: Type 2 #"(w620) -> ()
        n317 = global write "global1.vi" "1: Type 1"(w619) -> ()
        n318 = global write "global1.vi" "1: Type 2"(w611) -> ()
        n319 = global write "global1.vi" "2: Type 1"(w614) -> ()
        n320 = global write "global1.vi" "2: Type 2"(w610) -> ()
        n321 = global write "global1.vi" "3: Type 1"(w613) -> ()
        n322 = global write "global1.vi" "3: Type 2"(w609) -> ()
        n323 = global write "global1.vi" "4: Type 1"(w612) -> ()
        n324 = global write "global1.vi" "4: Type 2"(w608) -> ()
        n325 = global write "global1.vi" "Material 3"(w616) -> ()
        n326 = global write "global1.vi" "Material 4"(w615) -> ()
        n327 = global write "global1.vi" "Material 1"(w618) -> ()
        n328 = global write "global1.vi" "Material 2"(w617) -> ()
        n329 = Concatenate Strings(w618, w619) -> (w607:string)
        "1: Compound 1" <- w607
        n330 = Concatenate Strings(w617, w614) -> (w606:string)
        "2: Compound 1" <- w606
        n331 = Concatenate Strings(w616, w613) -> (w605:string)
        "3: Compound 1" <- w605
        n332 = Concatenate Strings(w615, w612) -> (w604:string)
        "4: Compound 1" <- w604
        n333 = Concatenate Strings(w618, w611) -> (w603:string)
        "1: Compoud 2" <- w603
        n334 = Concatenate Strings(w617, w610) -> (w602:string)
        "2: Compound 2" <- w602
        n335 = Concatenate Strings(w616, w609) -> (w601:string)
        "3: Compound 2" <- w601
        n336 = Concatenate Strings(w615, w608) -> (w600:string)
        "4: Compound 2" <- w600
        n337 = global write "global1.vi" "2: Compound 1"(w606) -> ()
        n338 = global write "global1.vi" "1: Compound 1"(w607) -> ()
        n339 = global write "global1.vi" "3: Compound 1"(w605) -> ()
        n340 = global write "global1.vi" "4: Compound 1"(w604) -> ()
        n341 = global write "global1.vi" "1: Compound 2"(w603) -> ()
        n342 = global write "global1.vi" "2: Compound 2"(w602) -> ()
        n343 = global write "global1.vi" "3: Compound 2"(w601) -> ()
        n344 = global write "global1.vi" "4: Compound 2"(w600) -> ()
        "Done with Phase One?" <- TRUE
      }
    }
    n345 = call-poly <vilib>:"PolyDisplay.vi"("Text"="Case #:  ", "NXT/EV3"=w18, "Line"=w15) -> ("NXT/EV3"=w17:T2)  [unwired: 1 in]
    n346 = call-poly <vilib>:"PolyDisplay.vi"("number"=w25, "NXT/EV3"=w17, "Line"=w24) -> ("NXT/EV3"=w8:T2)  [unwired: 1 in]
    n347 = call-poly <vilib>:"PolyWait.vi"("Time (1 sec)"=sgl 3.0, "NXT/EV3"=w8) -> ()  [unwired: 2 in, 1 out]
    n348 = local read "Done with Phase One?"() -> (w1:bool)
  }
